vi "getData.vi"(8 "error in (no error)":errorcluster, 11 "Instrument.VSource in":refnum<class "Instrument.VNA.lvclass">) -> (0 "error out":errorcluster, 2 "Data":variant, 3 "Instrument.VSource out":refnum<class "Instrument.VNA.lvclass">)   [LabVIEW 2019, in "Instrument.VNA.lvclass"]
uses:
  Instrument.VNA.lvclass
  C:/Users/patrick/Documents/GitHub/Instrument-Framework/lvsrc/Instrument/Instrument.lvclass
  7d887a1b-6fdf-430d-a3d5-06b059e03421.vi
  7d887a1b-6fdf-430d-a3d5-06b059e03421.vi/69b720f9-a455-49ef-b944-14bd92e8af79.vi
  7d887a1b-6fdf-430d-a3d5-06b059e03421.vi/69b720f9-a455-49ef-b944-14bd92e8af79.vi/26a7627e-a127-495f-8f45-2477aec6cb45.vi
  7d887a1b-6fdf-430d-a3d5-06b059e03421.vi/69b720f9-a455-49ef-b944-14bd92e8af79.vi/31ed9b66-b24c-4e02-8d33-b611e04fe8ce.vi
  Instrument/Private/Get RC Connection Status.vi
  Instrument/API/Send and Receive.vi
  <vilib>/Utility/Data Type/Get Type Information.vi
  <vilib>/JDP Science/JSONtext/JSON text to Variant.vi
  <vilib>/JDP Science/JSONtext/LVClass Serializer/JSONtext LVClass Serializer.lvclass
  Instrument/Instrument.lvclass
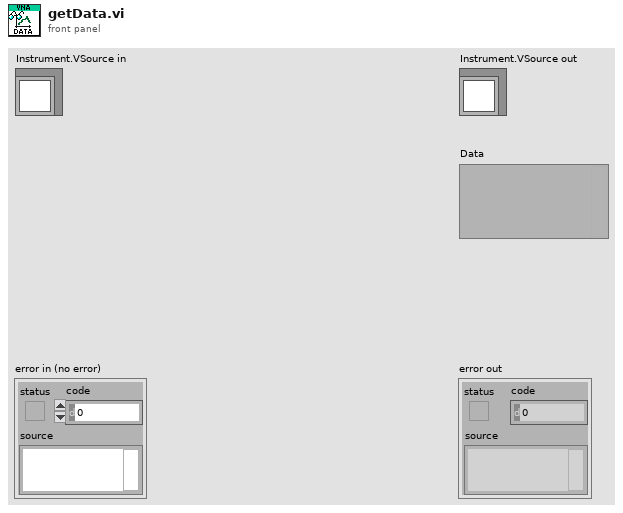
[diagram p1: front panel]
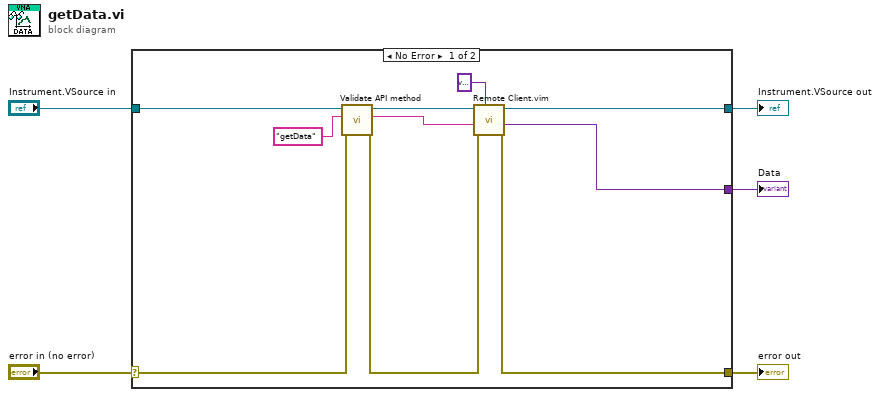
[diagram p0: block diagram]
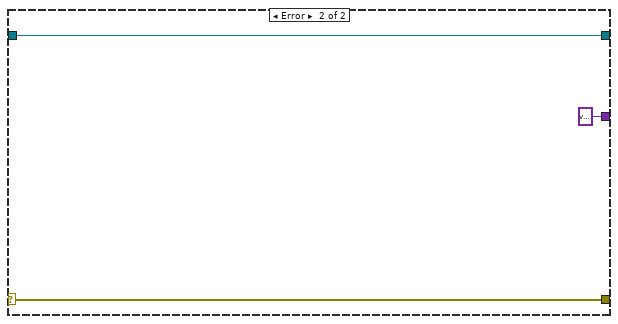
[diagram p2: hidden frame]
diagram:
  n1 = case shown="No Error" "error in (no error)" {
    selector: "error in (no error)" -> [w9 w18]
    tunnel: [w8 w18] -> w4
    tunnel: [w10 w17] -> w2
    tunnel: "Instrument.VSource in" -> [w12 w17]
    tunnel: [w11 variant ("Data out")] -> w1
    frame No Error {
      n2 = call "Validate API method.vi"("error in (no error)"=w9, "Command in"="getData" ("error message (\"\")"), "Instrument in"=w12) -> ("error out"=w7:errorcluster, "command out"=w6:string, "Instrument out"=w13:refnum<class "Instrument.VNA.lvclass">)  [unwired: 6 in]
      n3 = call "Remote Client.vim"("Data Out type"=variant, "error in (no error)"=w7, "Data in"=w6, "Instrument in"=w13) -> ("error out"=w8:errorcluster, "Data out"=w11:variant, "Instrument out"=w10:refnum<class "Instrument.VNA.lvclass">)  [unwired: 4 in, 1 out]
    }
    frame Error {
    }
  }
  "error out" <- w4
  "Instrument.VSource out" <- w2
  "Data" <- w1
